vi "generate filepath.vi"   [LabVIEW 2012]
uses:
  Custom Controls/file format type def.ctl
  GFG/GFGpathGet.vi
  GFG/GFGstringGet.vi
  GFG/GFG library.lvlib
types:
  T1 = typedef "file format type def.ctl" = enum16{"16bit raw", "32bit raw", "16bit multi-tiff (interleave)", "16bit multi-tiff (separate)", "16bit multi-tiff (stacked)", "32bit multi-tiff (interleave)", "32bit multi-tiff (separate)", "32bit multi-tiff (stacked)", "16bit tiff series (interleave)", "16bit tiff series (separate)", "16bit tiff series (stacked)", "32bit tiff series (interleave)", "32bit tiff series (separate)", "32bit tiff series (stacked)"}
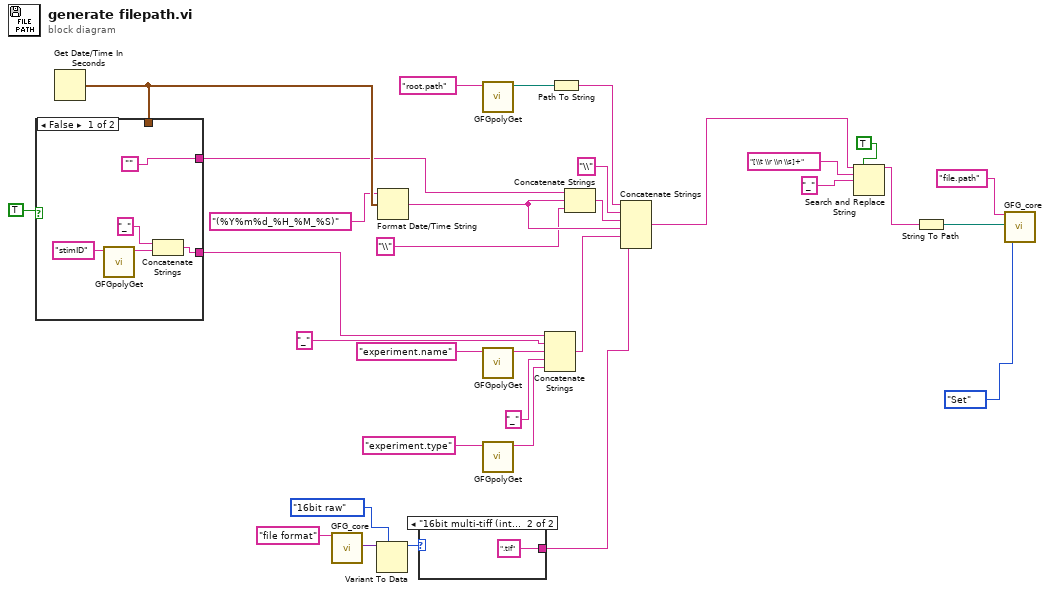
[diagram p0: block diagram]
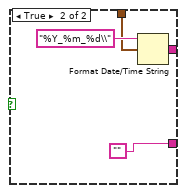
[diagram p2: hidden frame]
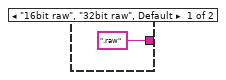
[diagram p3: hidden frame]
diagram:
  n1 = Get Date/Time In Seconds() -> (seconds since 1Jan1904=w32:timestamp)
  n2 = case shown="False" TRUE {
    tunnel: w32 -> [_ w40]
    tunnel: ["" w39] -> w29
    tunnel: [w33 ""] -> w3
    frame False {
      n3 = call-poly "GFGpolyGet.vi"("Variable Name in"="stimID") -> ("String"=w34:string)  [unwired: 10 in]
      n4 = Concatenate Strings("_" ("string"), w34) -> (w33:string)
    }
    frame True {
      n5 = Format Date/Time String(time format string (%c)="%Y_%m_%d\\", seconds (now)=w40) -> (date/time string=w39:string)  [unwired: 1 in]
    }
  }
  n6 = call "GFG_core.vi"("Variable Name in"="file format") -> ("Variant Out"=w21:variant)  [unwired: 12 in, 6 out]
  n7 = Variant To Data(type=file_format_type_def."16bit raw" ("file format"), Variant=w21) -> (data=w13:T1)  [unwired: 1 in, 1 out]
  n8 = Format Date/Time String(time format string (%c)="(%Y%m%d_%H_%M_%S)", seconds (now)=w32) -> (date/time string=w28:string)  [unwired: 1 in]
  n9 = case shown="\"16bit multi-tiff (interleave)\"..\"32bit tiff series (stacked)\"" w13 {
    tunnel: [".raw" ("string") ".tif" ("string")] -> w12
    frame "16bit raw", "32bit raw", Default {
    }
    frame "16bit multi-tiff (interleave)".."32bit tiff series (stacked)" {
    }
  }
  n10 = call-poly "GFGpolyGet.vi"("Variable Name in"="root.path") -> ("Path"=w26:path)  [unwired: 9 in, 1 out]
  n11 = call-poly "GFGpolyGet.vi"("Variable Name in"="experiment.name") -> ("String"=w17:string)  [unwired: 10 in]
  n12 = call-poly "GFGpolyGet.vi"("Variable Name in"="experiment.type") -> ("String"=w15:string)  [unwired: 10 in]
  n13 = Concatenate Strings(w3, "_" ("string"), w17, "_" ("string"), w15) -> (w14:string)
  n14 = Path To String(path=w26) -> (string=w18:string)
  n15 = Concatenate Strings(w29, w28, "\\" ("string")) -> (w31:string)
  n16 = Concatenate Strings(w18, "\\" ("string"), w31, w28, w14, w12) -> (w7:string)
  n17 = Search and Replace String(replace all?=TRUE ("replace all? (F)"), input string=w7, search string="[\\t \\r \\n \\s]+", replace string="_" ("replace string (\"\")")) -> (result string=w6:string)  [unwired: 4 in, 3 out]
  n18 = String To Path(string=w6) -> (path=w11:path)
  n19 = call "GFG_core.vi"("Variable Name in"="file.path" ("Tag in"), "Variant in"=w11, "Action"=enum16{"Init", "Set", "Get"}."Set") -> ()  [unwired: 10 in, 7 out]
